vi "ANSIshort.vi"() -> ()   [LabVIEW 2014]
doc: "This function doubles the value of input and returns the value in output.\n\nFor information on the data types used for the DLL function, right-click on the Call Library Function node and choose Configure."
uses:
  CLF_Example.dll
panel:
  out "output":i16
  in  "input":i16=10
  # "See the block diagram for more information."
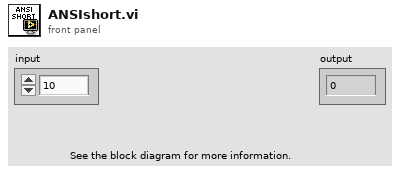
[diagram p1: front panel]
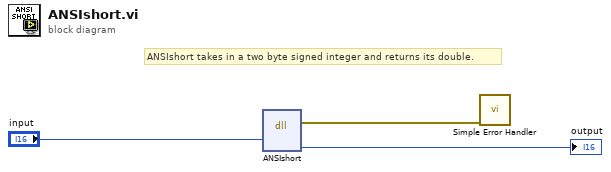
[diagram p0: block diagram]
diagram:
  # "ANSIshort takes in a two byte signed integer and returns its double."
  n1 = dll-call lib="e:/builds/penguin/labview/branches/2014/dev/dist/examples/Connectivity/Libraries and Executables/DLL Calling VIs/CLF_Example**.*" fn="ANSIshort"("input"="input") -> (error out=w1:errorcluster, "output"=→"output":i16)  [unwired: 4 in, 3 out]
  n2 = call <vilib>:"Simple Error Handler.vi"("error in (no error)"=w1) -> ()  [unwired: 4 in, 5 out]
